vi "Signal_acquisition_v3.vi"() -> ()   [LabVIEW 2015]
uses:
  <vilib>/measure/madcrms.llb/Basic Averaged DC-RMS for 1 Chan.vi
  <vilib>/measure/matone.llb/Extract Single Tone Information 1 Chan.vi
  <vilib>/express/express arith-compare/Formula/XNode/ExpressFormulaBlockNode.xnode
  <vilib>/measure/NI_MAPro.lvlib
panel:
  in  "timeout ms":i32=2000
  in  "timeout ms\n (2000)":i32=2000
  in  "timeout ms\n (2000) 2":i32=2000
  in  "Delay\n (# Samples)":i32 max=16348
  in  "Trigger Level \n(0 mV)":i32
  out "DC value 2":dbl format="%0.2p"
  out "detected \nfrequency 2":dbl format="%.2p"
  out "Ieration\nnumber":i32
  out "millisecond \ntimer value":u32
  out "millisecond \nbegin timer":u32
  out "millisecond \nfinal timer":u32
  in  "Tab Control":T1(tab)
  out "Voltage Gain / Frequency":cluster{i32, dbl}[](graph)
  out "Cutoff Freqs (Hz)":i32[](array[numeric])
  in  "MEASURE AMPLITUD":bool
  out "Acquisition\ntime complete":u32
  out "MEASURED \namplitud":dbl format="%.2p"
  out "RESULT \nin amplittude":dbl
  out "FRECUENCY \nEND":i32
  out "detected \nphase (deg)":dbl format="%.2p"
  out "detected \nfrequency":dbl format="%.2p"
  in  "Filename to save":path=path "test.lvm" caption="Filename"
  in  "Trigger Mode":string(combo)="CH1_NE"
  in  "input":u16=1
  in  "Pause \nfor buffer (ms)":u32=100
  out "error out":errorcluster
  in  "VOLTS":dbl=0.1
  in  "FREQ END":i32=70000
  in  "FREQ START":i32=10000
  in  "number \nof intervals":i32=60
  in  "IP address":string="161.111.10.6"
  in  "Decimation":u16(ring)=8 items=["65536"=65535, "8192"=8192, "1024"=1024, "64"=64, "16"=8, "1"=1]
  in  "error in":errorcluster
  out "REAL TIME MEASUREMENT":dbl[](graph)
  in  "FREQ START 5":i32
  in  "number of intervals  3":i32
  in  "number of intervals  2":i32
  # "FREQUENCY SWEEP"
  # "FREQUENCY SWEEP"
  # "Settings parameters"
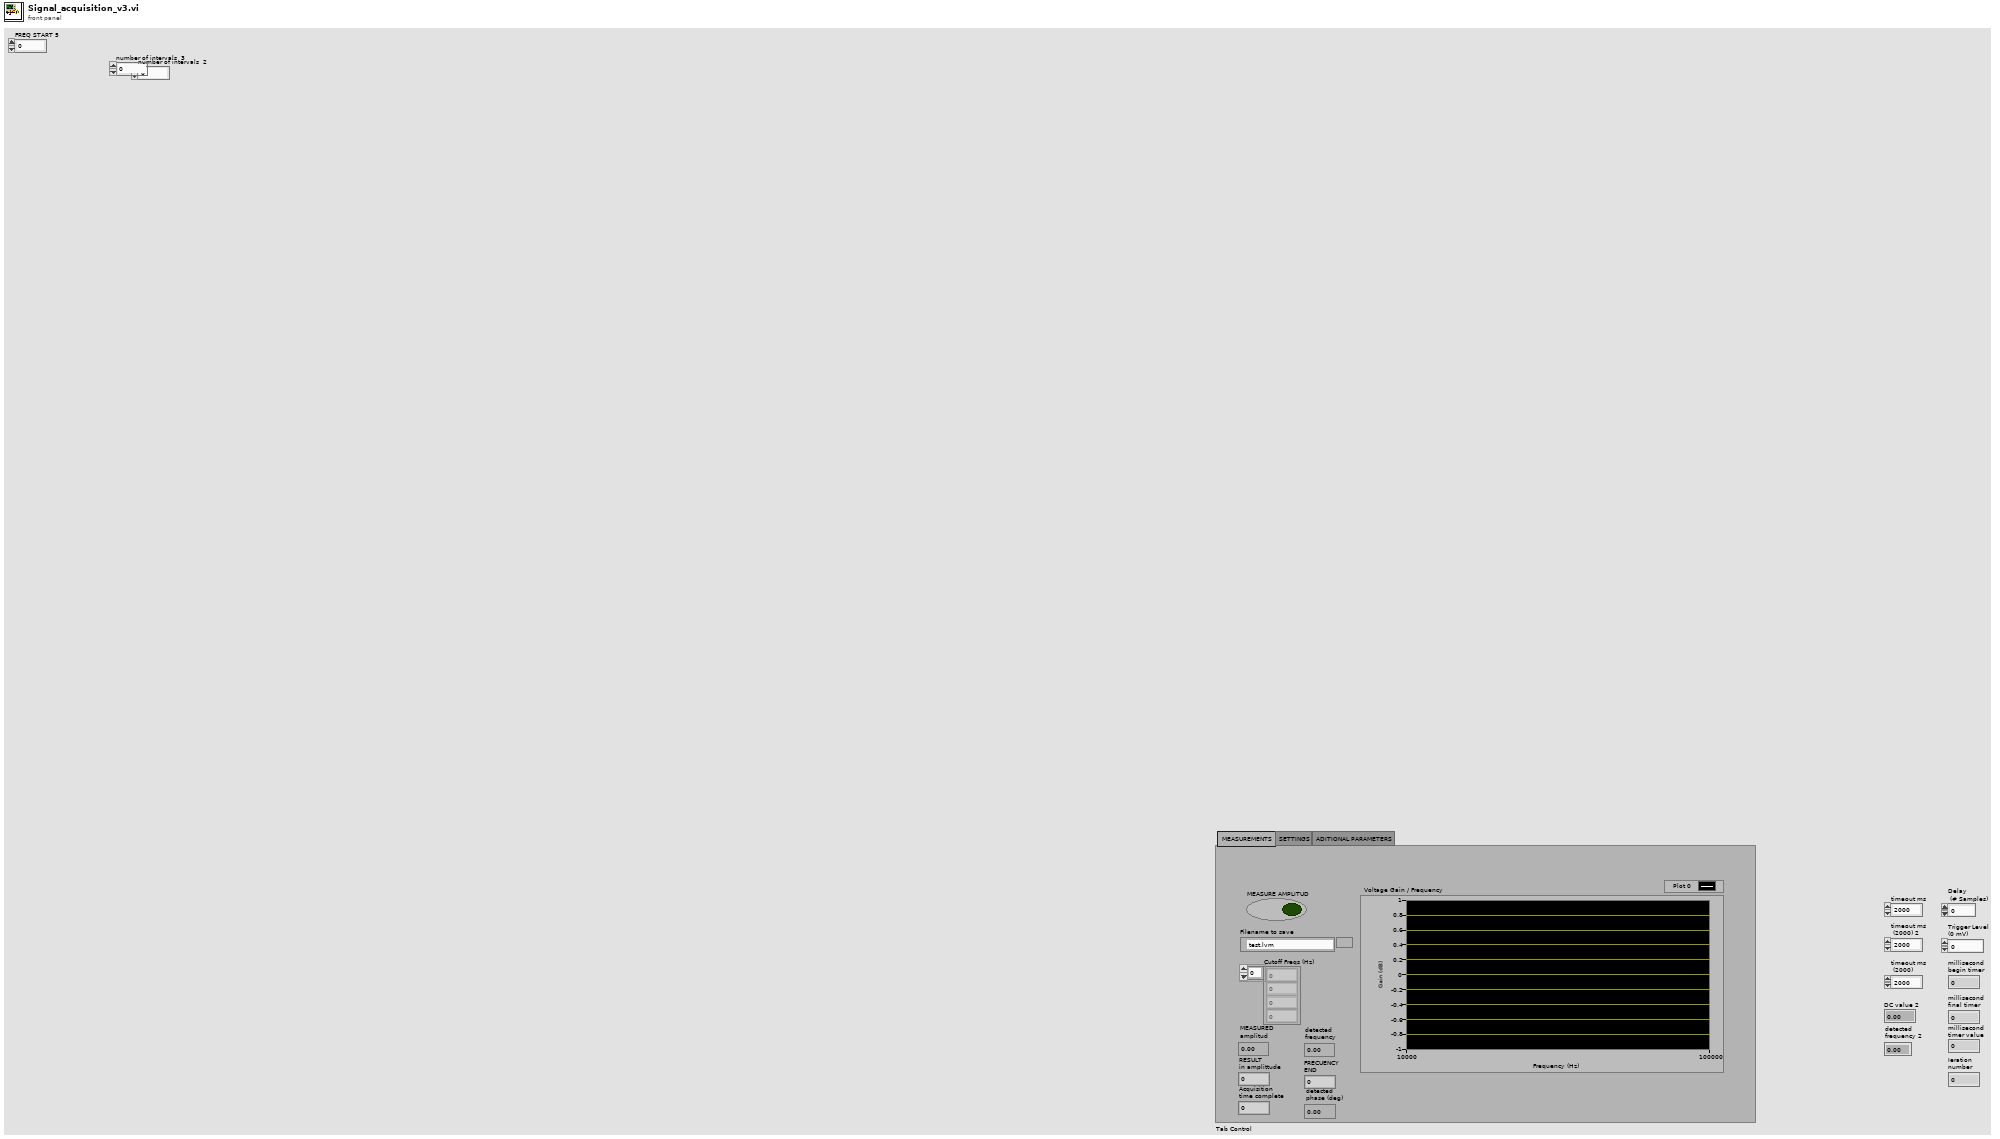
[diagram p1: front panel]
types:
  T1 = enum32{"MEASUREMENTS ", "SETTINGS", "ADITIONAL PARAMETERS"}
  T2 = enum16{"Standard", "Buffered", "CRLF", "Immediate"}
  T3 = enum32{"none", "input signal", "detected signal", "residual signal"}
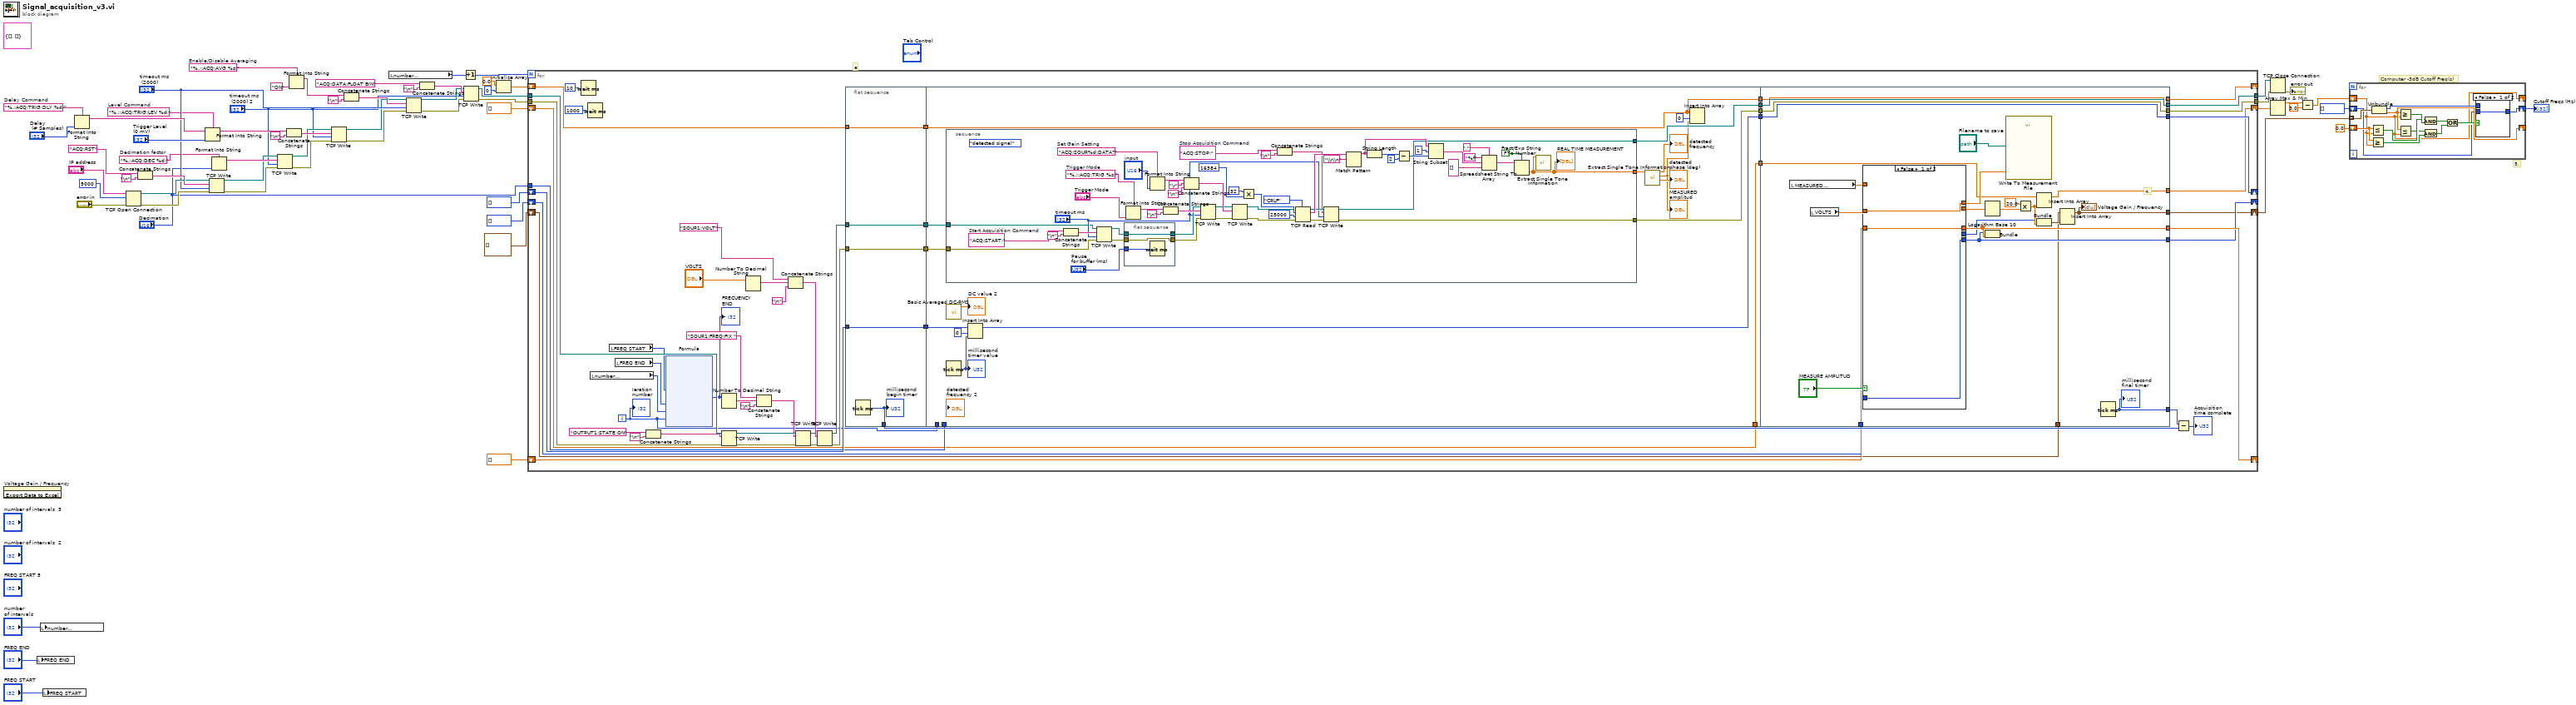
[diagram p0: block diagram]
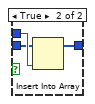
[diagram p2: hidden frame]
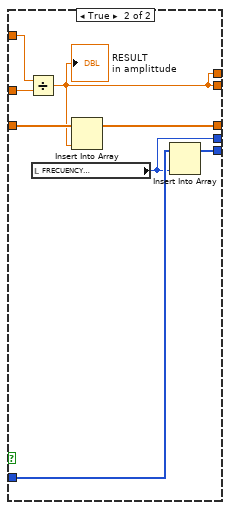
[diagram p3: hidden frame]
diagram:
  (unwired) cluster{dbl[], dbl[]} {[], []} ("FRECUENCY SWEEP")
  w29 = "%.;:ACQ:AVG %s;"  # Enable/Disable Averaging
  w37 = "%.;ACQ:DEC %d;"  # Decimation factor
  w38 = "%.;ACQ:TRIG:DLY %d;"  # Delay Command
  w39 = "%.;:ACQ:TRIG:LEV %d;"  # Level Command
  # "5."
  # "Computer -3dB Cutoff Freq(s)"
  # "e"
  n1 = invoke on="Voltage Gain / Frequency" class="XYGraph (strict)" method="Export Data to Excel"() -> ()  [unwired: 3 in, 3 out]
  n2 = local write "FREQ END"("FREQ END") -> ()
  n3 = local write "number \nof intervals"("number \nof intervals") -> ()
  n4 = local write "FREQ START"("FREQ START") -> ()
  n5 = Format Into String(format string=w38, "Delay\n (# Samples)") -> (resulting string=w57:string)  [unwired: 2 in, 1 out]
  n6 = TCP Open Connection(address="IP address", remote port or service name=u16 5000, error in (no error)="error in") -> (connection ID=w51:refnum<k5>, error out=w50:errorcluster)  [unwired: 2 in]
  n7 = Concatenate Strings("ACQ:RST" ("SCPI Message"), "\n") -> (w53:string)
  n8 = Format Into String(format string=w39, initial string=w57, "Trigger Level \n(0 mV)") -> (resulting string=w54:string)  [unwired: 1 in, 1 out]
  n9 = TCP Write(connection ID=w51, data in=w53, error in (no error)=w50, 9:"timeout ms\n (2000)") -> (connection ID out=w35:refnum<k5>, error out=w34:errorcluster)  [unwired: 1 out]
  n10 = Format Into String(format string=w37, "Decimation") -> (resulting string=w36:string)  [unwired: 2 in, 1 out]
  n11 = TCP Write(connection ID=w35, data in=w36, error in (no error)=w34, 9:"timeout ms\n (2000) 2") -> (connection ID out=w33:refnum<k5>, error out=w32:errorcluster)  [unwired: 1 out]
  n12 = Concatenate Strings(w54, "\n") -> (w48:string)
  n13 = Format Into String(format string=w29, "ON") -> (resulting string=w60:string)  [unwired: 2 in, 1 out]
  n14 = TCP Write(connection ID=w33, data in=w48, error in (no error)=w32, 9:"timeout ms\n (2000) 2") -> (connection ID out=w31:refnum<k5>, error out=w30:errorcluster)  [unwired: 1 out]
  n15 = Concatenate Strings(w60, "\n") -> (w49:string)
  n16 = local read "number \nof intervals"() -> (w15:i32)
  n17 = TCP Write(connection ID=w31, data in=w49, error in (no error)=w30, 9:"timeout ms\n (2000)") -> (connection ID out=w27:refnum<k5>, error out=w26:errorcluster)  [unwired: 1 out]
  n18 = Concatenate Strings("ACQ:DATA:FLOAT BIN" ("SCPI Message"), "\n") -> (w45:string)
  n19 = Increment(x=w15) -> (x+1=w14:i32)
  n20 = TCP Write(connection ID=w27, data in=w45, error in (no error)=w26, 9:"timeout ms\n (2000) 2") -> (connection ID out=w24:refnum<k5>, error out=w23:errorcluster)  [unwired: 1 out]
  n21 = Initialize Array(0.0 ("element"), 0 ("dimension size")) -> (w18:dbl[])
  n22 = for {
    N: w14 -> [_]
    tunnel: w24 -> [w88]
    tunnel: [w115] -> w44
    tunnel: [w114] -> w43
    tunnel: w23 -> [w85]
    shift-right: [w117] -> _
    shift-left: u32[] [] -> [w116]
    tunnel: "Decimation" -> [w104]
    shift-right: [w101] -> _
    shift-left: w18 -> [w99]
    shift-right: [w81] -> _
    shift-left: dbl[] [] -> [w82]
    shift-right: [w77] -> _
    shift-left: i32[] [] -> [w76]
    shift-right: [w71] -> w3
    shift-left: dbl[] [] -> [w69]
    shift-right: [w68] -> w2
    shift-left: cluster{"FRECUENCY END":i32, dbl}[] [] -> [w67]
    i -> [w75]
    n23 = Wait (ms)(milliseconds to wait=u32 10) -> ()  [unwired: 1 out]
    n24 = Wait (ms)(milliseconds to wait=u32 1000) -> ()  [unwired: 1 out]
    n25 = local read "number \nof intervals"() -> (w78:i32)
    n26 = local read "FREQ START"() -> (w79:i32)
    n27 = local read "FREQ END"() -> (w80:i32)
    n28 = Concatenate Strings("OUTPUT1:STATE ON" ("SCPI Message"), "\n") -> (w97:string)
    n29 = xnode "Formula"("Fin"=w79, "Fend"=w80, "Ninter"=w78, "i"=w75) -> ("Result"=w72:i32)  [unwired: 1 in, 1 out]
    "FRECUENCY \nEND" <- w72
    n30 = Number To Decimal String(number=w72) -> (decimal integer string=w83:string)  [unwired: 1 in]
    n31 = TCP Write(connection ID=w88, data in=w97, error in (no error)=w85) -> (connection ID out=w94:refnum<k5>, error out=w93:errorcluster)  [unwired: 1 in, 1 out]
    n32 = Number To Decimal String(number="VOLTS") -> (decimal integer string=w66:string)  [unwired: 1 in]
    n33 = Concatenate Strings("SOUR1:FREQ:FIX " ("SCPI Message"), w83, "\n") -> (w90:string)
    n34 = Concatenate Strings("SOUR1:VOLT" ("SCPI Message"), w66, "\n") -> (w89:string)
    n35 = TCP Write(connection ID=w94, data in=w90, error in (no error)=w93) -> (connection ID out=w74:refnum<k5>, error out=w73:errorcluster)  [unwired: 1 in, 1 out]
    n36 = TCP Write(connection ID=w74, data in=w89, error in (no error)=w73) -> (connection ID out=w87:refnum<k5>, error out=w86:errorcluster)  [unwired: 1 in, 1 out]
    n37 = flat-sequence {
      tunnel: w116 -> [w134]
      tunnel: w86 -> [w135]
      tunnel: w87 -> [w136]
      tunnel: [w136] -> w110
      tunnel: [w135] -> w109
      tunnel: [w134] -> w108
      tunnel: [w133] -> w106
      tunnel: [w132] -> w100
      tunnel: w99 -> [w132]
      tunnel: [w148] -> w113
      tunnel: [w146] -> w112
      tunnel: [w145] -> w111
      tunnel: w110 -> [w152]
      tunnel: w109 -> [w151]
      tunnel: w108 -> [w147]
      tunnel: w104 -> [_]
      tunnel: [w141] -> w102
      tunnel: w75 -> [_]
      tunnel: w100 -> [w141]
      tunnel: w69 -> [w137]
      tunnel: [w137] -> w70
      tunnel: [w229] -> w114
      tunnel: [w230] -> w115
      tunnel: [w231] -> w117
      tunnel: w113 -> [w231]
      tunnel: w112 -> [w230]
      tunnel: w111 -> [w229]
      tunnel: [w228] -> w107
      tunnel: w102 -> [w227]
      tunnel: [w227] -> w101
      tunnel: w82 -> [w223]
      tunnel: [w221] -> w81
      tunnel: [w220] -> w77
      tunnel: w76 -> [w222]
      tunnel: [w215] -> w71
      tunnel: w70 -> [w214]
      tunnel: [w212] -> w68
      tunnel: w67 -> [w211]
      frame #0 {
        n38 = Tick Count (ms)() -> (millisecond timer value=w133:u32)
        "millisecond \nbegin timer" <- w133
      }
      frame #1 {
        n39 = stacked-sequence {
          tunnel: w152 -> [w154]
          tunnel: w151 -> [w157]
          tunnel: [w155] -> w146
          tunnel: [w156] -> w145
          tunnel: [w153] -> w139
          frame #0 {
            w164 = "ACQ:STOP;"  # Stop Acquisition Command
            (unwired) T3."detected signal" ("export mode")
            w174 = "ACQ:SOUR%d:DATA?"  # Set Gain Setting
            w201 = "%.;:ACQ:TRIG %s;"  # Trigger Mode
            w203 = "ACQ:START;"  # Start Acquisition Command
            n40 = Concatenate Strings(w203, "\n") -> (w204:string)
            n41 = TCP Write(connection ID=w154, data in=w204, error in (no error)=w157, 9:"timeout ms") -> (connection ID out=w178:refnum<k5>, error out=w177:errorcluster)  [unwired: 1 out]
            n42 = flat-sequence {
              tunnel: "Pause \nfor buffer (ms)" -> [w207]
              tunnel: [w206] -> w176
              tunnel: [w205] -> w175
              tunnel: w178 -> [w206]
              tunnel: w177 -> [w205]
              frame #0 {
                n43 = Wait (ms)(milliseconds to wait=w207) -> ()  [unwired: 1 out]
              }
            }
            n44 = Format Into String(format string=w201, "Trigger Mode") -> (resulting string=w198:string)  [unwired: 2 in, 1 out]
            n45 = Format Into String(format string=w174, "input") -> (resulting string=w172:string)  [unwired: 2 in, 1 out]
            n46 = Concatenate Strings(w198, "\n") -> (w199:string)
            n47 = Concatenate Strings(w172, "\r", "\n") -> (w171:string)
            n48 = TCP Write(connection ID=w176, data in=w199, error in (no error)=w175, 9:"timeout ms") -> (connection ID out=w169:refnum<k5>, error out=w168:errorcluster)  [unwired: 1 out]
            n49 = TCP Write(connection ID=w169, data in=w171, error in (no error)=w168) -> (connection ID out=w170:refnum<k5>, error out=w167:errorcluster)  [unwired: 1 in, 1 out]
            n50 = Multiply(x=32, y=16384 ("bytes to read")) -> (x*y=w179:i32)
            n51 = Concatenate Strings(w164, "\n") -> (w162:string)
            n52 = TCP Read(connection ID=w170, bytes to read=w179, error in (no error)=w167, 7:T2."CRLF" ("mode (standard)"), 9:25000 ("timeout ms (25000)")) -> (connection ID out=w165:refnum<k5>, data out=w180:string, error out=w161:errorcluster)
            n53 = TCP Write(connection ID=w165, data in=w162, error in (no error)=w161, 9:"timeout ms") -> (connection ID out=w155:refnum<k5>, error out=w156:errorcluster)  [unwired: 1 out]
            n54 = Match Pattern(string=w180, regular expression="\\r\\n") -> (before substring=w186:string)  [unwired: 1 in, 3 out]
            n55 = String Length(string=w186) -> (length=w189:i32)
            n56 = Subtract(x=w189, y=2) -> (x-y=w190:i32)
            n57 = String Subset(string=w186, offset (0)=1, length (rest)=w190) -> (substring=w187:string)
            n58 = Spreadsheet String To Array(delimiter (Tab)=",", format string="%f", spreadsheet string=w187, array type (2D Dbl)=string[] [] ("Array")) -> (array=w193:string[])
            n59 = Fract/Exp String To Number(use system decimal point (T)=FALSE, string=w193) -> (number=w153:dbl[])  [unwired: 3 out]
            "REAL TIME MEASUREMENT" <- w153
            n60 = call-poly <vilib>:"Extract Single Tone Information.vi"("time signal in"=w153) -> ()  [unwired: 5 in, 6 out]
          }
        }
        n61 = call-poly <vilib>:"Basic Averaged DC-RMS.vi"() -> ("DC value"=→"DC value 2":dbl)  [unwired: 8 in, 3 out]
        n62 = Tick Count (ms)() -> (millisecond timer value=w149:u32)
        "millisecond \ntimer value" <- w149
        n63 = Insert Into Array(array=w147, index=0, new element=w149) -> (w148:u32[])
        n64 = call-poly <vilib>:"Extract Single Tone Information.vi"("time signal in"=w139) -> ("detected phase (deg)"=→"detected \nphase (deg)":dbl, "detected amplitude"=w138:dbl, "detected frequency"=→"detected \nfrequency":dbl)  [unwired: 5 in, 3 out]
        "MEASURED \namplitud" <- w138
        n65 = Insert Into Array(array=w141, index=0, new element=w138) -> ()  [unwired: 1 out]
      }
      frame #2 {
        # "4."
        n66 = local read "MEASURED \namplitud"() -> (w226:dbl)
        n67 = local read "VOLTS"() -> (w208:dbl)
        n68 = case shown="False" "MEASURE AMPLITUD" {
          tunnel: w226 -> [_ w238]
          tunnel: [w232 w237] -> w224
          tunnel: w223 -> [w234 w242]
          tunnel: [w234 w241] -> w221
          tunnel: [w233 w240] -> w220
          tunnel: w222 -> [w233 w239]
          tunnel: [_ w237] -> w210
          tunnel: [_ w236] -> w213
          tunnel: w208 -> [w232 w235]
          frame False {
          }
          frame True {
            n69 = Divide(x=w238, y=w235) -> (x/y=w237:dbl)
            "RESULT \nin amplittude" <- w237
            n70 = local read "FRECUENCY \nEND"() -> (w236:i32)
            n71 = Insert Into Array(array=w242, new element=w237) -> (w241:dbl[])  [unwired: 1 in]
            n72 = Insert Into Array(array=w239, new element=w236) -> (w240:i32[])  [unwired: 1 in]
          }
        }
        n73 = Logarithm Base 10(1:w210) -> (0:w217:dbl)
        n74 = Bundle(w220, w221) -> ()  [unwired: 1 in, 1 out]
        n75 = call "Write To Measurement File"("Signals"=w224, "Filename"="Filename to save") -> ()  [unwired: 15 in, 3 out]
        n76 = Multiply(x=20.0, y=w217) -> (x*y=w216:dbl)
        n77 = Insert Into Array(array=w214, new element=w216) -> (w215:dbl[])  [unwired: 1 in]
        n78 = Bundle("FRECUENCY \nEND"=w213, w216) -> (w219:cluster{"FRECUENCY \nEND":i32, dbl})  [unwired: 1 in]
        n79 = Insert Into Array(array=w211, new element=w219) -> (w212:cluster{"FRECUENCY END":i32, dbl}[])  [unwired: 1 in]
        "Voltage Gain / Frequency" <- w212
        n80 = Tick Count (ms)() -> (millisecond timer value=w228:u32)
        "millisecond \nfinal timer" <- w228
      }
    }
    n81 = Subtract(x=w107, y=w106) -> (x-y=→"Acquisition\ntime complete":u32)
    "Ieration\nnumber" <- w75
  }
  n82 = TCP Close Connection(connection ID=w44, error in (no error)=w43) -> (error out=→"error out":errorcluster)  [unwired: 1 in, 1 out]
  n83 = Array Max & Min(array=w3) -> (max value=w4:dbl)  [unwired: 3 out]
  n84 = Subtract(x=w4, y=3.0) -> (x-y=w5:dbl)
  n85 = for {
    tunnel: w2 -> [w256] mode=indexing
    shift-right: [w250] -> _
    shift-left: 0.0 -> [w251]
    shift-right: [w244] -> w7
    shift-left: i32[] [] -> [w245]
    shift-right: [w243] -> _
    shift-left: w5 -> [w243]
    n86 = Less Or Equal?(x=w251, y=w243) -> (x <= y?=w254:bool)
    n87 = Greater Or Equal?(x=w251, y=w243) -> (x >= y?=w252:bool)
    n88 = Unbundle(w256) -> ("FRECUENCY END"=w246:i32, w250:dbl)
    n89 = Greater Or Equal?(x=w250, y=w243) -> (x >= y?=w255:bool)
    n90 = Less Or Equal?(x=w250, y=w243) -> (x <= y?=w253:bool)
    n91 = And(x=w254, y=w255) -> (x .and. y?=w248:bool)
    n92 = And(x=w253, y=w252) -> (x .and. y?=w249:bool)
    n93 = Or(x=w248, y=w249) -> (x .or. y?=w247:bool)
    n94 = case shown="False" w247 {
      tunnel: w246 -> [_ w260]
      tunnel: w245 -> [w257 w259]
      tunnel: [w257 w258] -> w244
      frame False {
      }
      frame True {
        n95 = Insert Into Array(array=w259, new element=w260) -> (w258:i32[])  [unwired: 1 in]
      }
    }
  }
  "Cutoff Freqs (Hz)" <- w7
